vi "ViconL_Receiver.vi"() -> ()   [LabVIEW 2015]
uses:
  <vilib>/Utility/tcp.llb/UDP Multicast Read-Only Open.vi
panel:
  in  "Tab Control":enum32{"Charts"}(tab)
  out "Translation":dbl[][](graph)
  out "y":dbl
  out "z":dbl
  out "x":dbl
  in  "Stop":bool
  out "roll":dbl
  out "pitch":dbl
  out "yaw":dbl
  out "Rotation":dbl[][](graph)
  out "error out":errorcluster
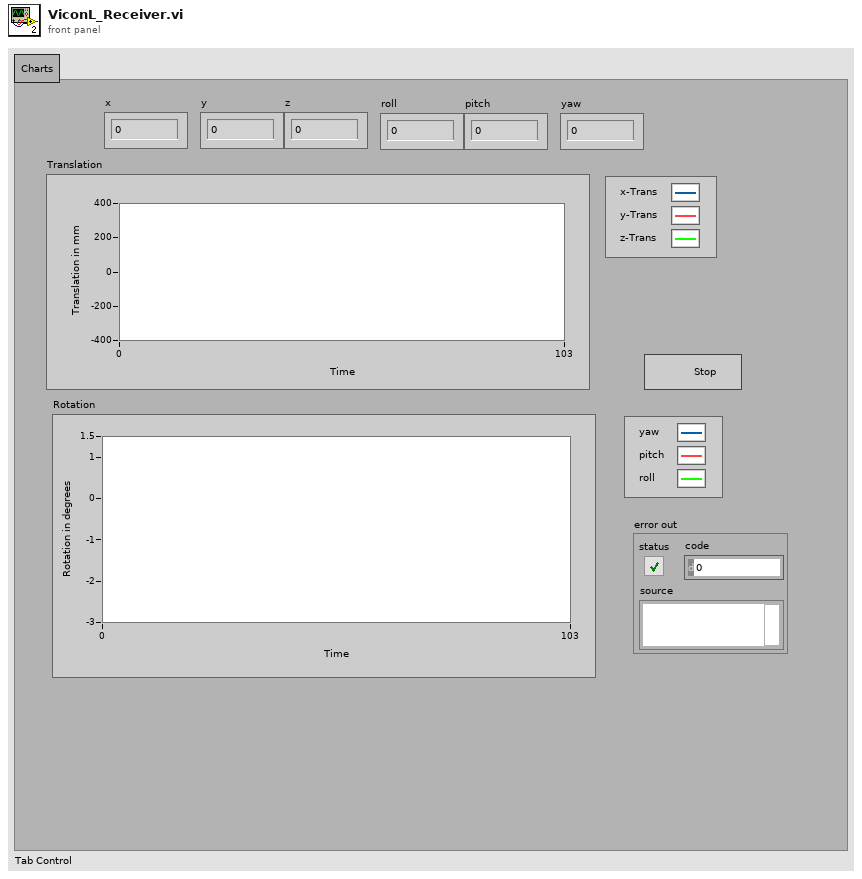
[diagram p1: front panel]
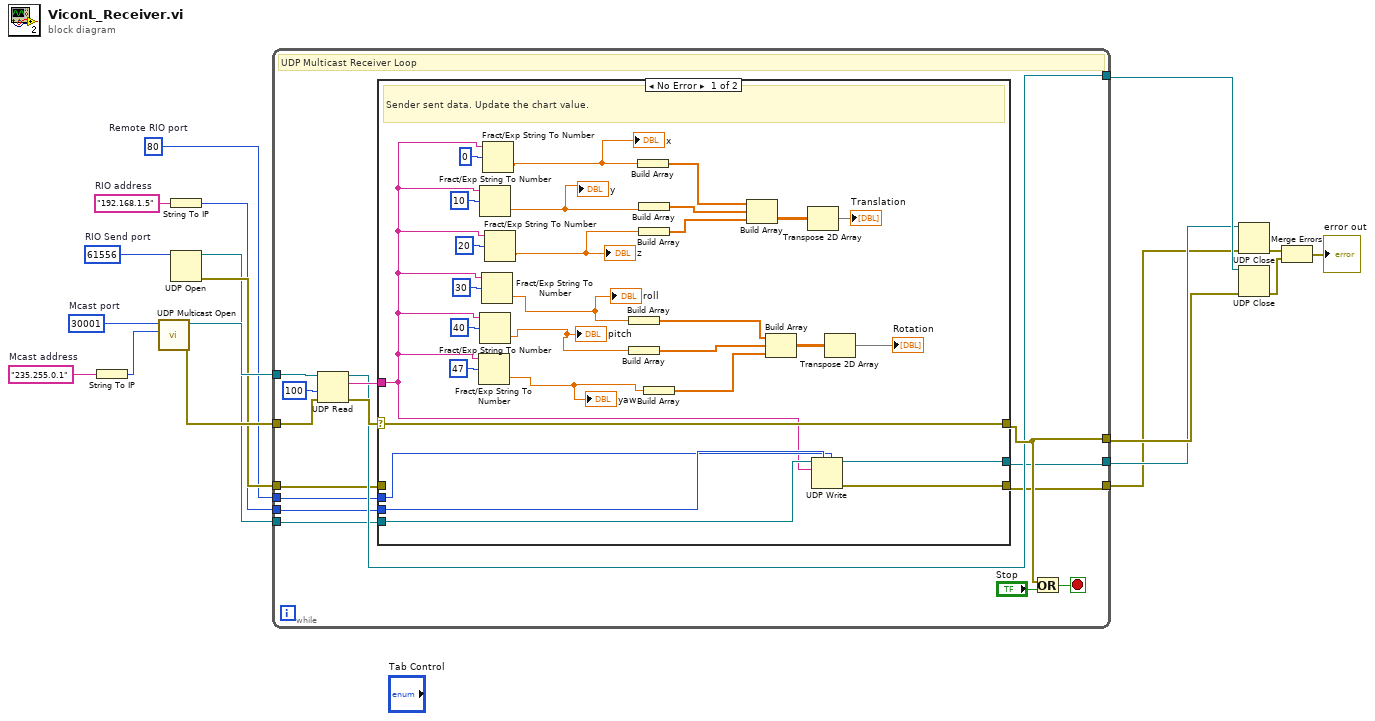
[diagram p0: block diagram]
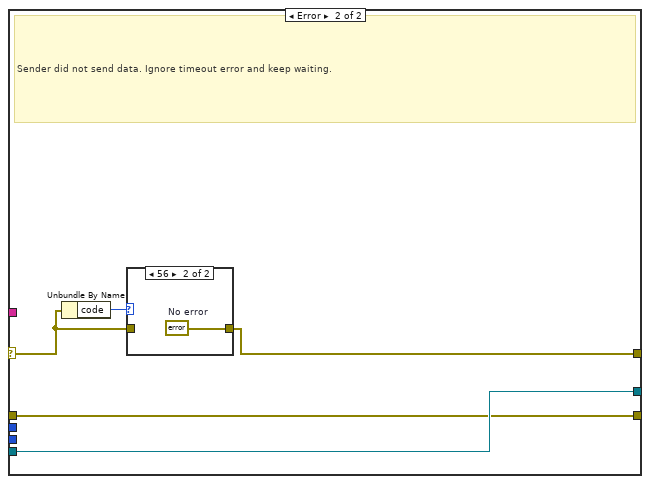
[diagram p2: hidden frame]
diagram:
  w6 = u16 80  # Remote RIO port
  w10 = u16 61556  # RIO Send port
  w11 = "192.168.1.5"  # RIO address
  w13 = u16 30001  # Mcast port
  w17 = "235.255.0.1"  # Mcast address
  n1 = String To IP(1:w17) -> (0:w12:u32)
  n2 = call-poly <vilib>:"UDP Multicast Open.vi"("multicast addr"=w12, "port"=w13) -> ("error out"=w15:errorcluster, "connection ID"=w14:refnum<k16>)  [unwired: 7 in, 1 out]
  n3 = String To IP(1:w11) -> (0:w7:u32)
  n4 = UDP Open(11:w10) -> (port=w8:refnum<k16>, 0:w9:errorcluster)  [unwired: 4 in, 1 out]
  n5 = while {
    tunnel: w14 -> [w33]
    tunnel: [w25] -> w18
    tunnel: w15 -> [w30]
    tunnel: [w26] -> w16
    tunnel: w9 -> [w19]
    tunnel: w8 -> [w24]
    tunnel: w7 -> [w23]
    tunnel: w6 -> [w22]
    tunnel: [w21] -> w5
    tunnel: [w20] -> w4
    stop <- w31 stop-if-true
    # "UDP Multicast Receiver Loop"
    n6 = UDP Read(connection ID=w33, timeout ms (25000)=100, 8:w30) -> (data out=w28:string, error out=w27:errorcluster, 3:w25:refnum<k16>)  [unwired: 3 out]
    n7 = case shown="No Error" w27 {
      selector: w27 -> [w57 w66]
      tunnel: w28 -> [w40 _]
      tunnel: [w57 w65] -> w26
      tunnel: w24 -> [w62 w64]
      tunnel: w23 -> [w61 _]
      tunnel: w22 -> [w60 _]
      tunnel: [w59 w64] -> w21
      tunnel: [w58 w63] -> w20
      tunnel: w19 -> [_ w63]
      frame No Error {
        # "Sender sent data. Update the chart value."
        n8 = Fract/Exp String To Number(string=w40, offset=47) -> (number=w35:dbl)  [unwired: 2 in, 1 out]
        "yaw" <- w35
        n9 = Fract/Exp String To Number(string=w40, offset=10) -> (number=w38:dbl)  [unwired: 2 in, 1 out]
        "y" <- w38
        n10 = Fract/Exp String To Number(string=w40, offset=40) -> (number=w34:dbl)  [unwired: 2 in, 1 out]
        "pitch" <- w34
        n11 = Fract/Exp String To Number(string=w40, offset=30) -> (number=w36:dbl)  [unwired: 2 in, 1 out]
        "roll" <- w36
        n12 = Fract/Exp String To Number(string=w40, offset=0) -> (number=w39:dbl)  [unwired: 2 in, 1 out]
        "x" <- w39
        n13 = Fract/Exp String To Number(string=w40, offset=20) -> (number=w37:dbl)  [unwired: 2 in, 1 out]
        "z" <- w37
        n14 = Build Array(w36) -> (w43:dbl[])
        n15 = Build Array(w34) -> (w44:dbl[])
        n16 = Build Array(w39) -> (w47:dbl[])
        n17 = Build Array(w38) -> (w46:dbl[])
        n18 = Build Array(w37) -> (w51:dbl[])
        n19 = Build Array(w35) -> (w45:dbl[])
        n20 = Build Array(w47, w46, w51) -> (w53:dbl[][])
        n21 = Build Array(w43, w44, w45) -> (w42:dbl[][])
        n22 = Transpose 2D Array(2D array=w53) -> (transposed array=→"Translation":dbl[][])
        n23 = UDP Write(address=w61, port or service name=w60, connection ID=w62, data in=w40) -> (error out=w58:errorcluster, 3:w59:refnum<k16>)  [unwired: 2 in]
        n24 = Transpose 2D Array(2D array=w42) -> (transposed array=→"Rotation":dbl[][])
      }
      frame Error {
        # "Sender did not send data. Ignore timeout error and keep waiting."
        n25 = Unbundle By Name(w66) -> ("code"=w67:i32)
        n26 = case shown="56" w67 {
          tunnel: w66 -> [w68 _]
          tunnel: [w68 w69] -> w65
          frame Default {
          }
          frame 56 {
            w69 = errorcluster {"status"=FALSE, "code"=0, "source"=""}  # No error
          }
        }
      }
    }
    n27 = Or(x=w26, y="Stop") -> (x .or. y?=w31:bool)
  }
  n28 = UDP Close(connection ID=w5, 8:w4) -> (error out=w3:errorcluster)  [unwired: 1 out]
  n29 = UDP Close(connection ID=w18, 8:w16) -> (error out=w2:errorcluster)  [unwired: 1 out]
  n30 = Merge Errors(w3, w2) -> (→"error out":errorcluster)
